vi "Teleop[Conflict].vi"(10 "Match Info":T1={"Autonomous Elapsed Seconds"=0.0, "TeleOp Elapsed Seconds"=0.0, "Disabled Elapsed Seconds"=0.0, "Visited Autonomous"=FALSE, "Visited TeleOp"=FALSE, "Visited Disabled"=FALSE, "Autonomous Settings"={"Autonomous Style"=enum."Independent", "VI Refnum"=refnum}}, 11 "Call Context":T2) -> ()   [LabVIEW 2017]
doc: "This VI is called for each TeleOp packet received from the DS where the robot is not disabled. It is often used to read from the joysticks and update I/O or to update setpoints for timed control loops. It should complete and return within 20 milliseconds or it may miss DS packets."
uses:
  <vilib>/Rock Robotics/WPI/DriverStation/WPI_DriverStationDerivedRobotMode.ctl
  <vilib>/Rock Robotics/WPI/DriverStation/WPI_DriverStationMatch Info.ctl
  <vilib>/Rock Robotics/WPI/Solenoid/WPI_SolenoidValue.ctl
  Public/Documents/Cross The Road Electronics/Phoenix-LabVIEW/Motor Controller/Controls/CTRE_Phoenix_MotorControl_ControlMode.ctl
  <vilib>/Rock Robotics/WPI/ThirdParty/Phoenix-LabVIEW/Motor Controller/Controls/CTRE_Phoenix_MotorControl_NeutralMode.ctl
  <vilib>/Rock Robotics/WPI/Utilities/WPI_GetSetVariantRefNum.vi
  <vilib>/Rock Robotics/Network Tables/NT Write Boolean Array.vi
  <vilib>/Rock Robotics/Network Tables/NT Write Numeric Array.vi
  <vilib>/Rock Robotics/Network Tables/NT Read Boolean.vi
  <vilib>/Rock Robotics/Network Tables/NT Read String.vi
  <vilib>/Rock Robotics/WPI/Joystick/WPI_JoystickArcadeMapping.vi
  <vilib>/Rock Robotics/Network Tables/NT Write Number.vi
  <vilib>/Rock Robotics/Network Tables/NT Read Numeric Array.vi
panel:
  out "String":string
  out "element":dbl
  in  "L Retract Ramps":bool
  in  "R Retract Ramps":bool
  in  "RRamp Raise":bool
  in  "LRamp Raise":bool=TRUE
  in  "RRamp Deploy":bool
  in  "LRamp Deploy":bool
  in  "Cube Down":bool
  in  "Cube Up":bool
  in  "Direction Toggle":bool
  in  "Gear Shift":bool
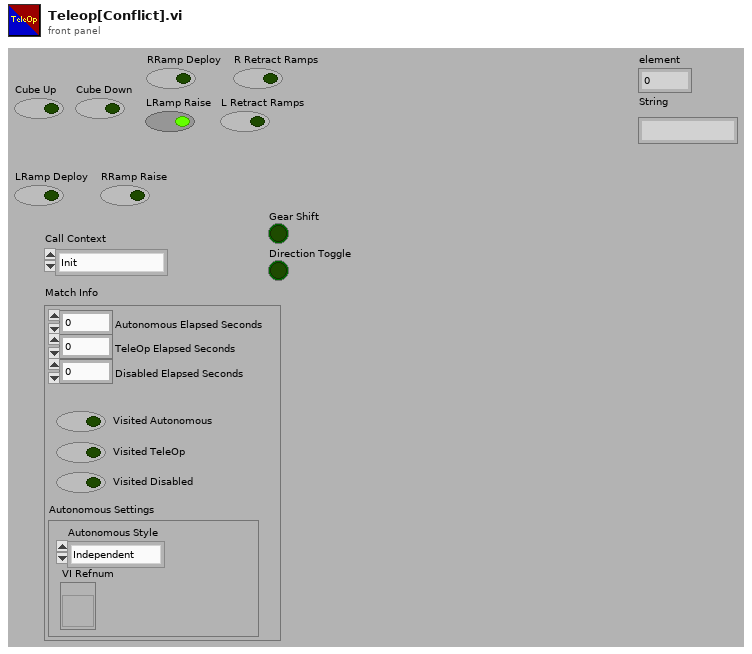
[diagram p1: front panel]
types:
  T1 = typedef "WPI_DriverStationMatch Info.ctl" = cluster{"Autonomous Elapsed Seconds":dbl, "TeleOp Elapsed Seconds":dbl, "Disabled Elapsed Seconds":dbl, "Visited Autonomous":bool, "Visited TeleOp":bool, "Visited Disabled":bool, "Autonomous Settings":cluster{"Autonomous Style":enum16{"Iterative", "Independent"}, "VI Refnum":refnum<vi>}}
  T2 = typedef "WPI_DriverStationDerivedRobotMode.ctl" = enum16{"Init", "Execute", "Stop"}
  T3 = typedef "CTRE_Phoenix_MotorControl_NeutralMode.ctl" = enum8{"EEPROMSetting", "Override to Coast", "Override to Brake"}
  T4 = typedef "CTRE_Phoenix_MotorControl_ControlMode.ctl" = u16
  T5 = typedef "WPI_SolenoidValue.ctl" = enum16{"Off", "On", "Forward", "Reverse"}
  T6 = typedef "WPI_JoystickDevRef.ctl" = cluster{"Device":T7}
  T7 = typedef "WPI_JoystickDeviceEnum.ctl" = enum16{"USB 0", "USB 1", "USB 2", "USB 3", "USB 4", "USB 5"}
  T8 = typedef "WPI_MotorControlDeviceRef.ctl" = cluster{"DeviceStatus":errorcluster, "Type":T9, "PWM":cluster{"PWM Channel":T10, "DeadBand":T11}, "CAN":cluster{"Device Number":u8, "SetOutput VI Ref":variant, "GetOutput VI Ref":variant, "Enable VI Ref":variant, "Disable VI Ref":variant, "Data":variant}, "Invert":bool, "DIO PWM":cluster{"PWM \"Enable\" Channel":T10, "DIOChannel":T12, "PWM Rate":dbl}}
  T9 = typedef "WPI_MotorControlType.ctl" = enum16{"PWM", "CAN", "DIO PWM"}
  T10 = typedef "FPGA_DIOPWMChannel.ctl" = enum8{"PWM 0", "PWM 1", "PWM 2", "PWM 3", "PWM 4", "PWM 5", "PWM 6", "PWM 7", "PWM 8", "PWM 9", "PWM MXP 0", "PWM MXP 1", "PWM MXP 2", "PWM MXP 3", "PWM MXP 4", "PWM MXP 5", "PWM MXP 6", "PWM MXP 7", "PWM MXP 8", "PWM MXP 9", "Invalid"}
  T11 = typedef "WPI_PWMDeadband.ctl" = cluster{"Name":string, "maxPositivePwm":i32, "minPositivePwm":i32, "centerPwm":i32, "maxNegativePwm":i32, "minNegativePwm":i32, "angularRange":u16}
  T12 = typedef "FPGA_DIOChannel.ctl" = enum8{"DIO 0", "DIO 1", "DIO 2", "DIO 3", "DIO 4", "DIO 5", "DIO 6", "DIO 7", "DIO 8", "DIO 9", "DIO MXP 0", "DIO MXP 1", "DIO MXP 2", "DIO MXP 3", "DIO MXP 4", "DIO MXP 5", "DIO MXP 6", "DIO MXP 7", "DIO MXP 8", "DIO MXP 9", "DIO MXP 10", "DIO MXP 11", "DIO MXP 12", "DIO MXP 13", "DIO MXP 14", "DIO MXP 15", "SPI Port CS1", "SPI Port CS2", "SPI Port CS3", "SPI Port MISO", "SPI Port MOSI", "Invalid"}
  T13 = typedef "WPI_SolenoidDevRef.ctl" = cluster{"DevStatus":errorcluster, "Pneumatics Control Module":u8, "Forward Solenoid Channel":T14, "Reverse Solenoid Channel":T14}
  T14 = typedef "WPI_SolenoidChannel.ctl" = enum8{"Solenoid 0", "Solenoid 1", "Solenoid 2", "Solenoid 3", "Solenoid 4", "Solenoid 5", "Solenoid 6", "Solenoid 7", "Invalid"}
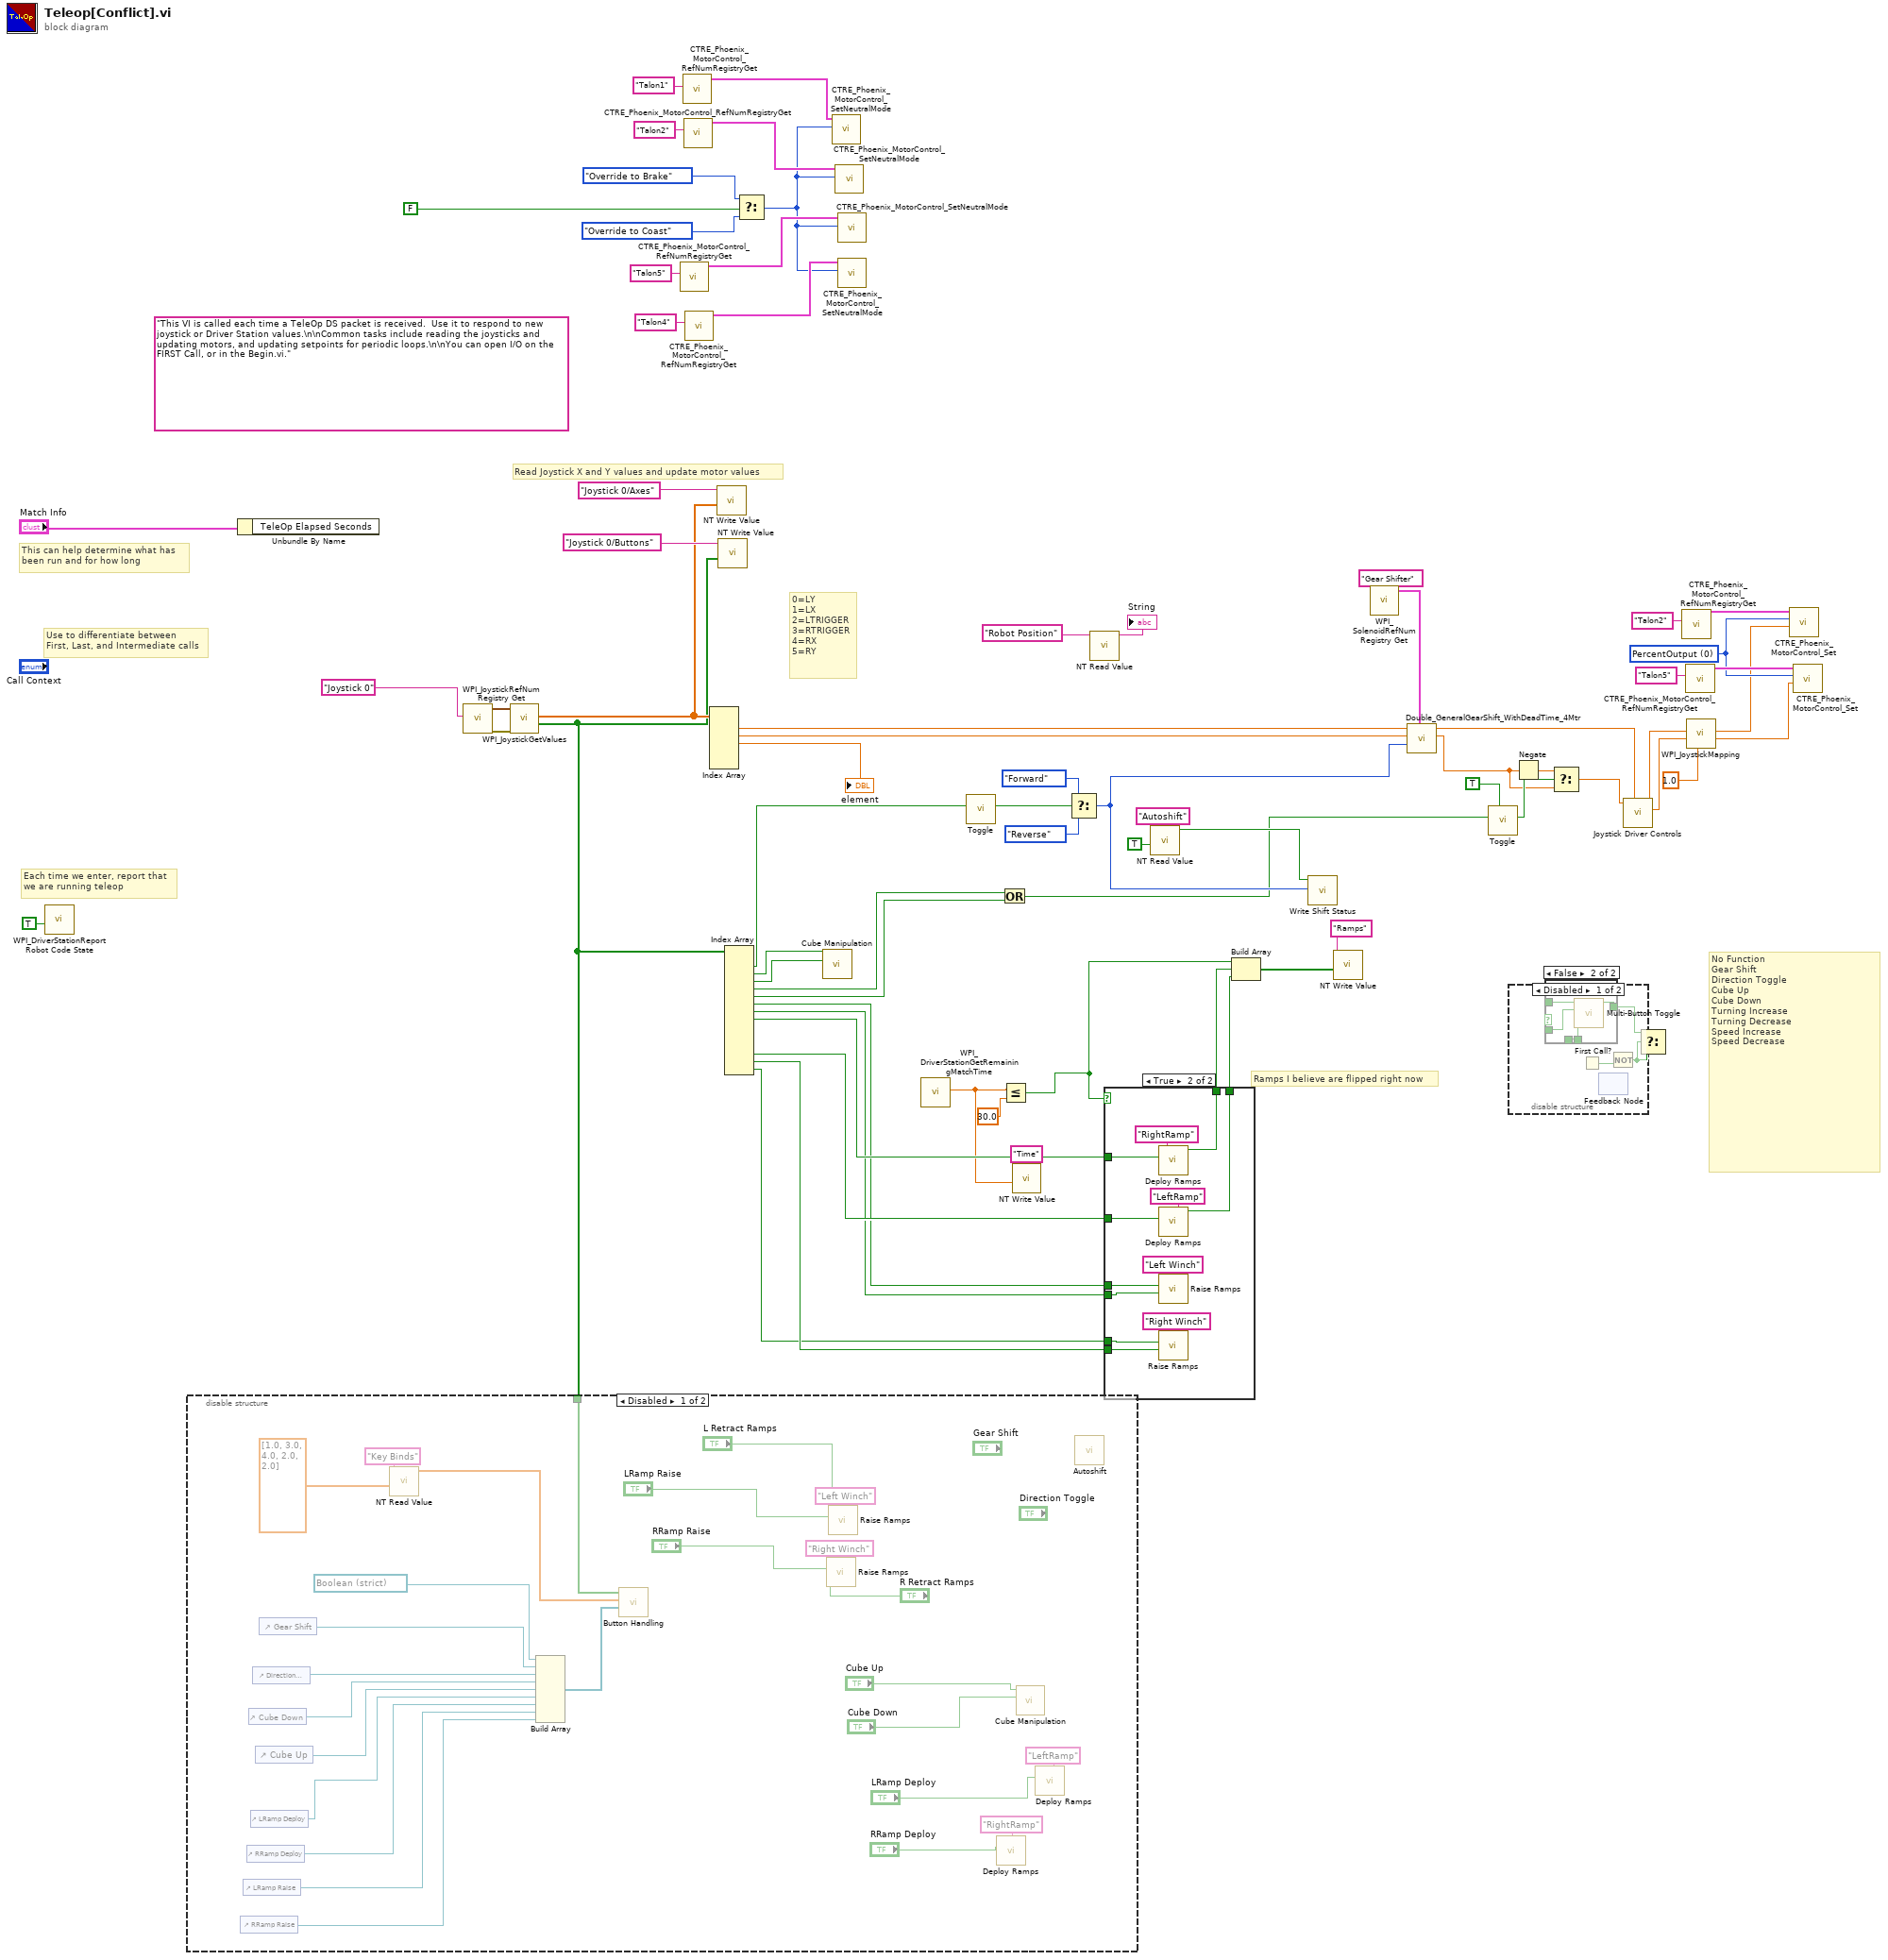
[diagram p0: block diagram]
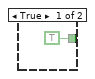
[diagram p2: hidden frame]
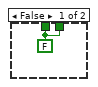
[diagram p4: hidden frame]
diagram:
  w34 = T4 0 items=["PercentOutput"=0, "Position"=1, "Velocity"=2, "Current"=3, "Follower"=5, "MotionProfile"=6, "MotionMagic"=7, "MotionMagicArc"=8, "MotionProfileArc"=10, "Disabled"=15] ("Control Mode")
  (unwired) "This VI is called each time a TeleOp DS packet is received.  Use it to respond to new joystick or Driver Station values.\n\nCommon tasks include reading the joysticks and updating motors, and updating setpoints for periodic loops.\n\nYou can open I/O on the FIRST Call, or in the Begin.vi."
  # "Ramps I believe are flipped right now"
  # "No Function\nGear Shift\nDirection Toggle\nCube Up\nCube Down\nTurning Increase\nTurning Decrease\nSpeed Increase\nSpeed Decrease"
  # "0=LY\n1=LX\n2=LTRIGGER\n3=RTRIGGER\n4=RX\n5=RY"
  # "Each time we enter, report that\nwe are running teleop"
  # "Use to differentiate between\nFirst, Last, and Intermediate calls"
  # "This can help determine what has\nbeen run and for how long"
  # "Read Joystick X and Y values and update motor values"
  n1 = call <vilib>:"WPI_DriverStationReport Robot Code State.vi"("TeleOp"=TRUE ("Autonomous")) -> ()  [unwired: 10 in, 1 out]
  n2 = Unbundle By Name("Match Info") -> ()  [unwired: 1 out]
  n3 = call <vilib>:"WPI_JoystickRefNum Registry Get.vi"("refnum name"="Joystick 0") -> ("error out"=w56:errorcluster, "JoystickDevRef"=w70:T6)  [unwired: 1 in, 8 out]
  n4 = call <vilib>:"WPI_JoystickGetValues.vi"("error in (no error)"=w56, "JoystickDevRef"=w70) -> ("Buttons"=w55:bool[], "Axes"=w66:dbl[])  [unwired: 5 in, 3 out]
  n5 = disable-structure shown="Disabled" {
    disable-tunnel: w55 -> [w74 _]
    frame Disabled {
      n6 = control-ref of="RRamp Raise"() -> (w88:refnum<vi>)
      n7 = control-ref of="LRamp Raise"() -> (w89:refnum<vi>)
      n8 = control-ref of="RRamp Deploy"() -> (w91:refnum<vi>)
      n9 = control-ref of="Cube Down"() -> (w94:refnum<vi>)
      n10 = control-ref of="LRamp Deploy"() -> (w92:refnum<vi>)
      n11 = control-ref of="Direction Toggle"() -> (w96:refnum<vi>)
      n12 = control-ref of="Cube Up"() -> (w93:refnum<vi>)
      n13 = control-ref of="Gear Shift"() -> (w97:refnum<vi>)
      n14 = call-poly <vilib>:"NT Read Value.vi"("Default Value"=dbl[] [1.0, 3.0, 4.0, 2.0, 2.0], "Name"="Key Binds") -> ("Numeric Array"=w73:dbl[])  [unwired: 8 in, 1 out]
      n15 = Build Array(refnum<vi> refnum ("element"), w97, w96, w94, w93, w92, w91, w89, w88) -> (w72:refnum<vi>[])
      n16 = call "Button Handling.vi"("Array"=w72, "Numeric Array"=w73, "Buttons"=w74) -> ()  [unwired: 9 in]
      n17 = call "Raise Ramps.vi"("Retract Ramps"="R Retract Ramps", "Raise Ramps"="RRamp Raise", "refnum name"="Right Winch") -> ()  [unwired: 9 in]
      n18 = call "Raise Ramps.vi"("Retract Ramps"="L Retract Ramps", "Raise Ramps"="LRamp Raise", "refnum name"="Left Winch") -> ()  [unwired: 9 in]
      n19 = call "Deploy Ramps.vi"("Deploy"="RRamp Deploy", "refnum name"="RightRamp") -> ()  [unwired: 9 in, 1 out]
      n20 = call "Cube Manipulation.vi"("Outtake"="Cube Down", "Intake"="Cube Up") -> ()  [unwired: 10 in]
      n21 = call "Deploy Ramps.vi"("Deploy"="LRamp Deploy", "refnum name"="LeftRamp") -> ()  [unwired: 9 in, 1 out]
      n22 = call "Autoshift.vi"() -> ()  [unwired: 12 in]
    }
    frame Enabled {
    }
  }
  n23 = call "CTRE_Phoenix_MotorControl_RefNumRegistryGet.vi"("refnum name"="Talon5") -> ("PhoenixMotorControlDevRef"=w13:T8)  [unwired: 9 in, 1 out]
  n24 = call "CTRE_Phoenix_MotorControl_RefNumRegistryGet.vi"("refnum name"="Talon1") -> ("PhoenixMotorControlDevRef"=w6:T8)  [unwired: 9 in, 1 out]
  n25 = call "CTRE_Phoenix_MotorControl_RefNumRegistryGet.vi"("refnum name"="Talon2") -> ("PhoenixMotorControlDevRef"=w14:T8)  [unwired: 9 in, 1 out]
  n26 = call "CTRE_Phoenix_MotorControl_RefNumRegistryGet.vi"("refnum name"="Talon4") -> ("PhoenixMotorControlDevRef"=w8:T8)  [unwired: 9 in, 1 out]
  n27 = Index Array(array=w66) -> (element #1=w65:dbl, element #2=w64:dbl, element #3=→"element":dbl)  [unwired: 6 in, 3 out]
  n28 = call-poly <vilib>:"NT Write Value.vi"("Numeric Array"=w66, "Name"="Joystick 0/Axes") -> ()  [unwired: 9 in, 1 out]
  n29 = call-poly <vilib>:"NT Write Value.vi"("Boolean Array"=w55, "Name"="Joystick 0/Buttons") -> ()  [unwired: 9 in, 1 out]
  n30 = Index Array(array=w55) -> (element #1=w47:bool, element #2=w48:bool, element #3=w49:bool, element #4=w40:bool, element #5=w41:bool, element #6=w5:bool, element #7=w4:bool, element #8=w30:bool, element #9=w31:bool, element #10=w3:bool, element #11=w2:bool)  [unwired: 15 in, 4 out]
  n31 = Select(t=CTRE_Phoenix_MotorControl_NeutralMode."Override to Brake" ("Motor Control Neutral Mode"), s=FALSE, f=CTRE_Phoenix_MotorControl_NeutralMode."Override to Coast" ("Motor Control Neutral Mode")) -> (s? t:f=w7:T3)
  n32 = call "Cube Manipulation.vi"("Outtake"=w49, "Intake"=w48) -> ()  [unwired: 10 in]
  n33 = call <vilib>:"CTRE_Phoenix_MotorControl_SetNeutralMode.vi"("Motor Control Neutral Mode"=w7, "PhoenixMotorControlDevRef"=w6) -> ()  [unwired: 8 in, 2 out]
  n34 = call <vilib>:"CTRE_Phoenix_MotorControl_SetNeutralMode.vi"("Motor Control Neutral Mode"=w7, "PhoenixMotorControlDevRef"=w14) -> ()  [unwired: 8 in, 2 out]
  n35 = call <vilib>:"CTRE_Phoenix_MotorControl_SetNeutralMode.vi"("Motor Control Neutral Mode"=w7, "PhoenixMotorControlDevRef"=w13) -> ()  [unwired: 8 in, 2 out]
  n36 = call <vilib>:"CTRE_Phoenix_MotorControl_SetNeutralMode.vi"("Motor Control Neutral Mode"=w7, "PhoenixMotorControlDevRef"=w8) -> ()  [unwired: 8 in, 2 out]
  n37 = call <vilib>:"WPI_DriverStationGetRemainingMatchTime.vi"() -> ("Match Time(s)"=w24:sgl)  [unwired: 10 in, 1 out]
  n38 = call "Toggle.vi"("Input"=w47) -> ("Output"=w62:bool)  [unwired: 10 in]
  n39 = Or(x=w40, y=w41) -> (x .or. y?=w42:bool)
  n40 = Less Or Equal?(x=w24, y=sgl 30.0) -> (x <= y?=w1:bool)
  n41 = call-poly <vilib>:"NT Write Value.vi"("Numeric"=w24, "Name"="Time") -> ()  [unwired: 9 in, 1 out]
  n42 = Select(t=WPI_SolenoidValue."Forward" ("Shift Value"), s=w62, f=WPI_SolenoidValue."Reverse" ("Shift Value")) -> (s? t:f=w46:T5)
  n43 = call-poly <vilib>:"NT Read Value.vi"("Name"="Robot Position") -> ("String"=→"String":string)  [unwired: 9 in, 1 out]
  n44 = case shown="True" w1 {
    tunnel: w5 -> [_ w106]
    tunnel: w4 -> [_ w105]
    tunnel: w30 -> [_ w104]
    tunnel: w31 -> [_ w103]
    tunnel: w3 -> [_ w102]
    tunnel: w2 -> [_ w101]
    tunnel: [w98 w100] -> w27
    tunnel: [w98 w99] -> w26
    frame False {
      w98 = FALSE ("Output")
    }
    frame True {
      n45 = call "Deploy Ramps.vi"("Deploy"=w104, "refnum name"="RightRamp") -> ("Output"=w100:bool)  [unwired: 9 in]
      n46 = call "Deploy Ramps.vi"("Deploy"=w103, "refnum name"="LeftRamp") -> ("Output"=w99:bool)  [unwired: 9 in]
      n47 = call "Raise Ramps.vi"("Retract Ramps"=w105, "Raise Ramps"=w106, "refnum name"="Left Winch") -> ()  [unwired: 9 in]
      n48 = call "Raise Ramps.vi"("Retract Ramps"=w102, "Raise Ramps"=w101, "refnum name"="Right Winch") -> ()  [unwired: 9 in]
    }
  }
  n49 = call-poly <vilib>:"NT Read Value.vi"("Default Value"=TRUE, "Name"="Autoshift") -> ("Boolean"=w43:bool)  [unwired: 8 in, 1 out]
  n50 = Build Array(w1, w27, w26) -> (w29:bool[])
  n51 = call "Write Shift Status.vi"("Gear"=w46, "Autoshifting"=w43) -> ()  [unwired: 9 in, 1 out]
  n52 = call-poly <vilib>:"NT Write Value.vi"("Boolean Array"=w29, "Name"="Ramps") -> ()  [unwired: 9 in, 1 out]
  n53 = call <vilib>:"WPI_SolenoidRefNum Registry Get.vi"("refnum name"="Gear Shifter") -> ("SolenoidDevRef"=w59:T13)  [unwired: 9 in, 1 out]
  n54 = call "Double_GeneralGearShift_WithDeadTime_4Mtr.vi"("ShifterRef"=w59, "Shift Value"=w46, "Right"=w64, "Left"=w65) -> ("Right Output"=w22:dbl, "Left Output"=w20:dbl)  [unwired: 4 in, 2 out]
  n55 = call "Toggle.vi"("Control"=TRUE, "Input"=w42) -> ("Output"=w54:bool)  [unwired: 9 in]
  n56 = disable-structure shown="Disabled" {
    frame Disabled {
      n57 = case shown="False" w115 {
        tunnel: [TRUE ("Output") w125] -> w112
        tunnel: [_ w124] -> w119
        tunnel: [_ w123] -> w118
        tunnel: [_ w122] -> w117
        tunnel: [_ w121] -> w116
        frame True {
        }
        frame False {
          n58 = call "Multi-Button Toggle.vi"("Button 4"=w121, "Button 3"=w122, "Button 2"=w123, "Button 1"=w124) -> ("Output"=w125:bool)  [unwired: 7 in]
        }
      }
      n59 = First Call?() -> (First Call?: T/F=w114:bool)
      n60 = feedback #1() -> ()  [unwired: 2 in]
      n61 = feedback-in #1() -> (w111)
      n62 = Not(x=w114) -> (.not. x?=w113:bool)
      n63 = Select(t=w112, s=w113, f=w113) -> ()  [unwired: 1 out]
    }
    frame Enabled {
    }
  }
  n64 = Negate(x=w22) -> (-x=w53:dbl)
  n65 = Select(t=w53, s=w54, f=w22) -> (s? t:f=w21:dbl)
  n66 = call "Joystick Driver Controls.vi"("X"=w20, "Y"=w21) -> ("Y"=w18:dbl, "X"=w19:dbl)  [unwired: 8 in]
  n67 = call "CTRE_Phoenix_MotorControl_RefNumRegistryGet.vi"("refnum name"="Talon2") -> ("PhoenixMotorControlDevRef"=w36:T8)  [unwired: 9 in, 1 out]
  n68 = call "CTRE_Phoenix_MotorControl_RefNumRegistryGet.vi"("refnum name"="Talon5") -> ("PhoenixMotorControlDevRef"=w35:T8)  [unwired: 9 in, 1 out]
  n69 = call-poly <vilib>:"WPI_JoystickMapping.vi"("Max Output"=1.0, "Y axis value"=w18, "X axis value"=w19) -> ("Right Motor Value"=w33:dbl, "Left Motor Value"=w32:dbl)  [unwired: 7 in]
  n70 = call <vilib>:"CTRE_Phoenix_MotorControl_Set.vi"("Output"=w32, "Control Mode"=w34, "PhoenixMotorControlDevRef"=w36) -> ()  [unwired: 7 in, 2 out]
  n71 = call <vilib>:"CTRE_Phoenix_MotorControl_Set.vi"("Output"=w33, "Control Mode"=w34, "PhoenixMotorControlDevRef"=w35) -> ()  [unwired: 7 in, 2 out]
